vi "Get System Settings.vi"(8 "error in (no error)":errorcluster, 11 "Config Data":T3) -> (0 "error out":errorcluster, 3 "System_Settings":T1)   [LabVIEW 2026, in "Acquisition.lvlib"]
uses:
  Acquisition.lvlib
  Controls/Options.ctl
  Controls/System_Settings.ctl
  Controls/Vibration_Monitor_Config.ctl
  Controls/Vibration_Profile.ctl
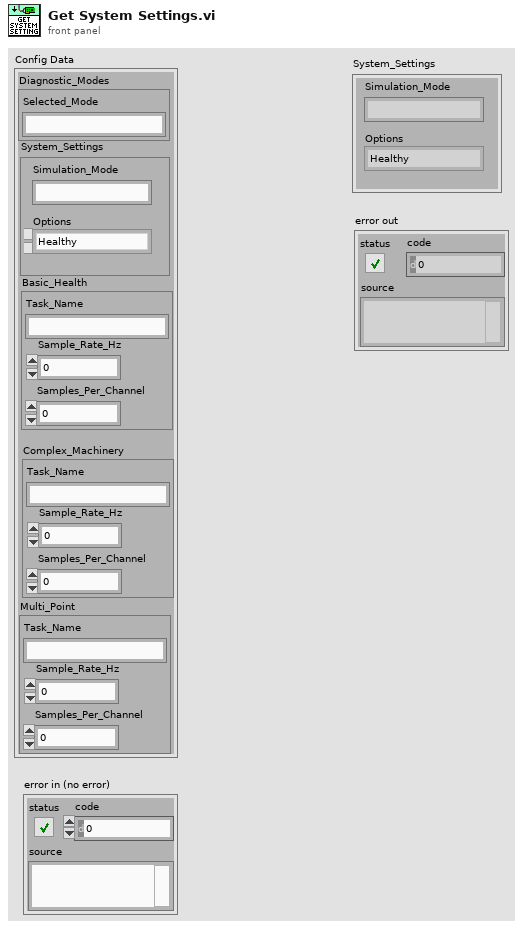
[diagram p1: front panel]
types:
  T1 = typedef "System_Settings.ctl" = cluster{"Simulation_Mode ":string, "Options":T2}
  T2 = typedef "Options.ctl" = enum16{"Healthy", "Unbalance_Alert", "Bearing_Fault_Critical", "Sweep_Test"}
  T3 = typedef "Vibration_Monitor_Config.ctl" = cluster{"Diagnostic_Modes":cluster{"Selected_Mode":string}, "Basic_Health":T4, "Complex_Machinery":T4, "Multi_Point":T4, "System_Settings":T1}
  T4 = typedef "Vibration_Profile.ctl" = cluster{"Task_Name":string, "Sample_Rate_Hz":dbl, "Samples_Per_Channel":i32}
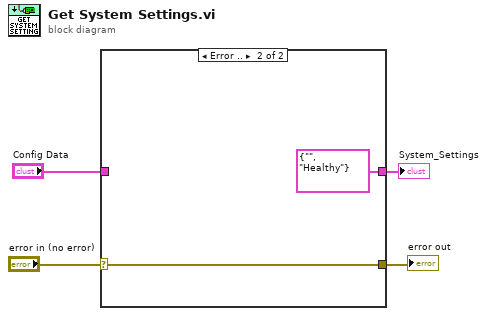
[diagram p0: block diagram]
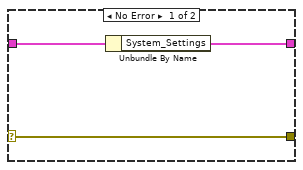
[diagram p2: hidden frame]
diagram:
  n1 = case shown="Error .." "error in (no error)" {
    selector: "error in (no error)" -> [w7 w9]
    tunnel: [w7 w9] -> w3
    tunnel: "Config Data" -> [w6 _]
    tunnel: [w5 T1 {"Simulation_Mode "="", "Options"=enum."Healthy"} ("System_Settings")] -> w1
    frame No Error {
      n2 = Unbundle By Name(w6) -> ("System_Settings"=w5:T1)
    }
    frame Error {
    }
  }
  "error out" <- w3
  "System_Settings" <- w1
